vi "VSSSpeedTransformation.vi"(10 "V_ang in":dbl, 11 "V_tang in":dbl) -> (2 "V_rigth":dbl, 3 "V_left":dbl)   [LabVIEW 2023]
panel:
  in  "K":dbl=1.0
  in  "Upper_limit":dbl=4.0
  in  "Robot_radius":dbl=0.05
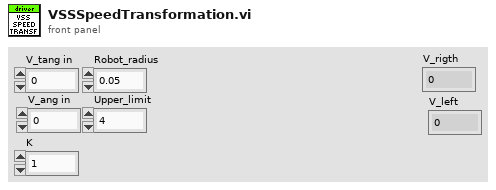
[diagram p1: front panel]
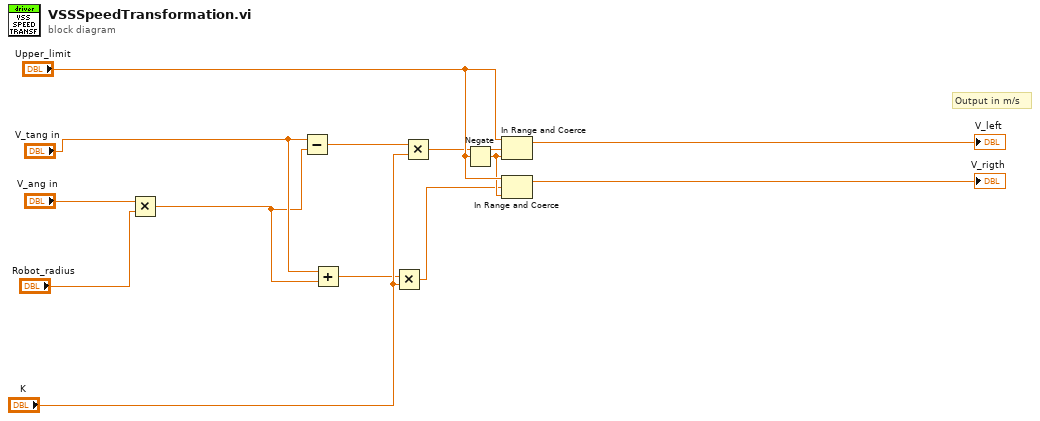
[diagram p0: block diagram]
diagram:
  # "Output in m/s"
  n1 = Multiply(x="V_ang in", y="Robot_radius") -> (x*y=w3:dbl)
  n2 = Subtract(x="V_tang in", y=w3) -> (x-y=w10:dbl)
  n3 = Add(x="V_tang in", y=w3) -> (x+y=w9:dbl)
  n4 = Multiply(x=w9, y="K") -> (x*y=w4:dbl)
  n5 = Multiply(x=w10, y="K") -> (x*y=w5:dbl)
  n6 = Negate(x="Upper_limit") -> (-x=w6:dbl)
  n7 = In Range and Coerce(upper limit="Upper_limit", x=w5, lower limit=w6) -> (coerced(x)=→"V_left":dbl)  [unwired: 1 out]
  n8 = In Range and Coerce(upper limit="Upper_limit", x=w4, lower limit=w6) -> (coerced(x)=→"V_rigth":dbl)  [unwired: 1 out]
